vi "Read Pot.vi"(8 "error in (no error)":errorcluster, 11 "MCP4018 Digipot In":refnum<class "MCP4018 Digipot.lvclass">) -> (0 "error out":errorcluster, 2 "Pot Value(0-127)":u8, 3 "MCP4018 Digipot out":refnum<class "MCP4018 Digipot.lvclass">)   [LabVIEW 2020, in "CTI-Peripheral.lvlib" / "MCP4018 Digipot.lvclass"]
uses:
  MCP4018 Digipot.lvclass
  MCP4018 Digipot.lvclass/MCP4018 Digipot.ctl
  CTI/I2C Connection/I2C Connection.lvclass/I2C Connection.ctl
  CTI/Session/I2C Read Data.vi
  CTI/I2C Connection/I2C Connection.lvclass
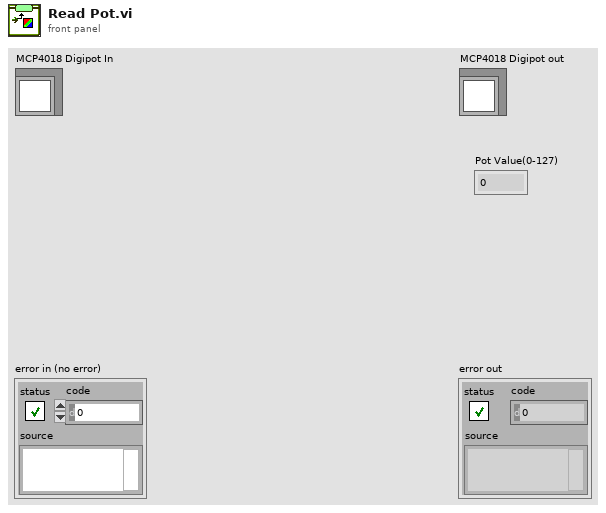
[diagram p1: front panel]
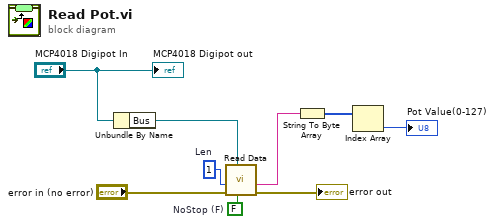
[diagram p0: block diagram]
diagram:
  w8 = FALSE  # NoStop (F)
  w9 = u8 1  # Len
  n1 = Unbundle By Name("MCP4018 Digipot In") -> ("Bus"=w7:refnum<class "I2C Connection.lvclass">)
  n2 = call "Read Data.vi"("NoStop (F)"=w8, "I2C Connection"=w7, "error in (no error)"="error in (no error)", "Len"=w9) -> ("error out"=→"error out":errorcluster, "Data"=w6:string)  [unwired: 6 in]
  n3 = String To Byte Array(string=w6) -> (unsigned byte array=w5:u8[])
  n4 = Index Array(array=w5) -> (element=→"Pot Value(0-127)":u8)  [unwired: 1 in]
  "MCP4018 Digipot out" <- "MCP4018 Digipot In"
